vi "Verify AND Parameterized.vi"(8 "error in":errorcluster) -> (0 "error out":errorcluster)   [LabVIEW 2020, in "Caraya Extension Tests.lvclass"]
uses:
  Caraya Extension Tests.lvclass
  <vilib>/addons/_JKI Toolkits/Caraya/classes/Test/Test.lvclass
  Source/Extensions/Caraya.Extension/Caraya.Extension.lvlib
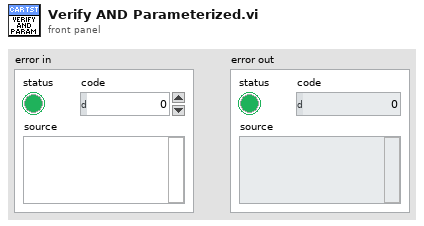
[diagram p1: front panel]
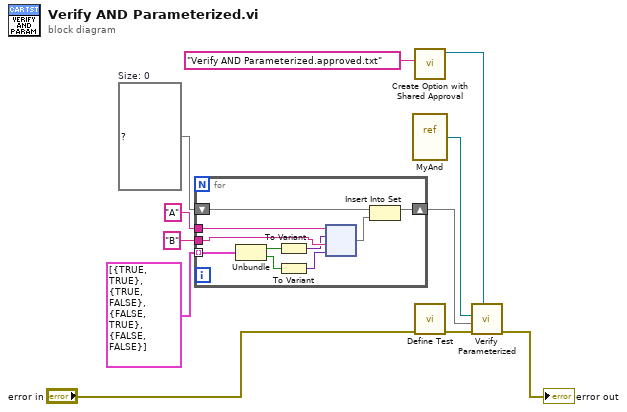
[diagram p0: block diagram]
diagram:
  w4 = set{map{string, variant}} {}  # Size: 0
  n1 = for {
    tunnel: "A" -> [w21]
    tunnel: cluster{bool, bool}[] [{TRUE, TRUE}, {TRUE, FALSE}, {FALSE, TRUE}, {FALSE, FALSE}] -> [w19] mode=indexing
    tunnel: "B" -> [w20]
    shift-right: [w13] -> w3
    shift-left: w4 -> [w12]
    n2 = Unbundle(w19) -> (w18:bool, w17:bool)
    n3 = To Variant(anything=w18) -> (Variant=w15:variant)
    n4 = To Variant(anything=w17) -> (Variant=w14:variant)
    n5 = node ("Build Map")(w21, w15, w20, w14) -> (w16:map{string, variant})
    n6 = Insert Into Set(10:w16, 11:w12) -> (3:w13:set{map{string, variant}})  [unwired: 1 out]
  }
  n7 = vi-ref "MyAnd.vi"() -> (w8:refnum<vi>)
  n8 = call "Create Option with Shared Approval.vi"("Filename"="Verify AND Parameterized.approved.txt") -> ("Options outs"=w1:refnum<class "Options.lvclass">)  [unwired: 10 in]
  n9 = call <vilib>:"Define Test.vi"("error in (no error)"="error in") -> ("error out"=w11:errorcluster)  [unwired: 9 in, 1 out]
  n10 = call "Verify Parameterized.vi"("Approvals"=w1, "error in"=w11, "ctl label -> value var"=w3, "VI Refnum"=w8) -> ("error out"=→"error out":errorcluster)  [unwired: 6 in, 1 out]
